vi "niRFUtil MEAS Max and Min (complex wfm).vi"(2 "Waveform In":T1 {"y" format="%.2f"; "dx" format="%^.2e"; "x0" format="%^.2e"}) -> (6 "Max":csg format="%.2f", 7 "Min":csg format="%.2f")   [LabVIEW 2015, in "niRFUtil.lvlib"]
doc: "(c) Copyright 2006, National Instruments, Inc. This VI may not be duplicated, sold, or distributed without written consent from National Instruments."
uses:
  niRFUtil.lvlib
  Includes/niRFUtil INC Complex Waveform.ctl
  Includes/niRFUtil INC Complex Array.ctl
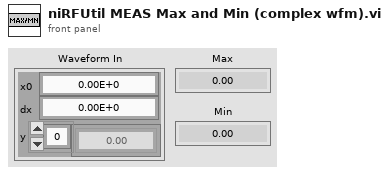
[diagram p1: front panel]
types:
  T1 = typedef "niRFUtil.lvlib/niRFUtil INC Complex Waveform.ctl" = cluster{"x0":dbl, "dx":dbl, "y":T2}
  T2 = typedef "niRFUtil.lvlib/niRFUtil INC Complex Array.ctl" = csg[]
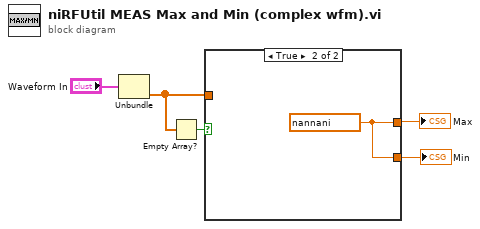
[diagram p0: block diagram]
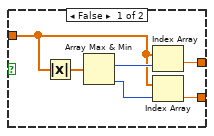
[diagram p2: hidden frame]
diagram:
  n1 = Unbundle("Waveform In") -> ("y"=w1:T2)  [unwired: 2 out]
  n2 = Empty Array?(array=w1) -> (empty?=w2:bool)
  n3 = case shown="True" w2 {
    tunnel: [w9 w12] -> w4
    tunnel: w1 -> [w7 _]
    tunnel: [w6 w12] -> w3
    frame False {
      n4 = Absolute Value(x=w7) -> (abs(x)=w11:sgl[])
      n5 = Array Max & Min(array=w11) -> (max index (indices)=w10:i32, min index (indices)=w8:i32)  [unwired: 2 out]
      n6 = Index Array(array=w7, index=w10) -> (element=w9:csg)
      n7 = Index Array(array=w7, index=w8) -> (element=w6:csg)
    }
    frame True {
      w12 = csg nan+nani ("Numeric")
    }
  }
  "Max" <- w4
  "Min" <- w3
